vi "Box Colour FGV.vi"(8 "error in (no error)":errorcluster, 10 "Colour to detect":T1=enum."Black", 11 "Init/R/W State":T2) -> (0 "error out":errorcluster, 3 "Colour to detect (output)":T1)   [LabVIEW 2018]
uses:
  Box Colour FGV States.ctl
  Box Colour FGV Colours.ctl
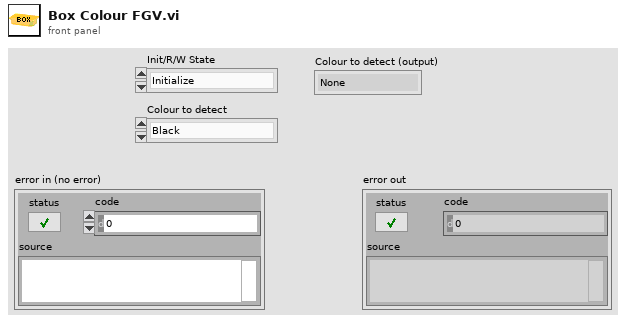
[diagram p1: front panel]
types:
  T1 = typedef "Box Colour FGV Colours.ctl" = enum16{"None", "Black", "Blue", "Green", "Red", "Yellow"}
  T2 = typedef "Box Colour FGV States.ctl" = enum16{"Initialize", "Read", "Write"}
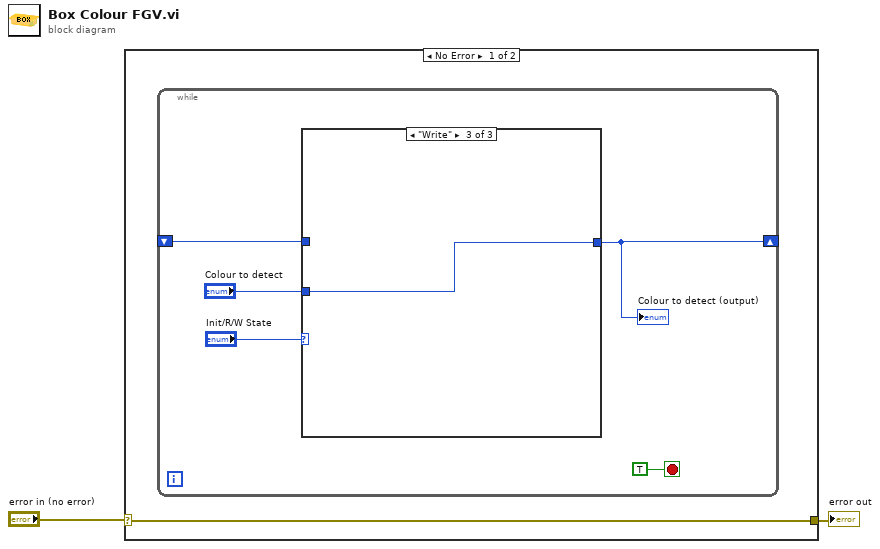
[diagram p0: block diagram]
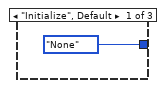
[diagram p2: hidden frame]
diagram:
  n1 = case shown="No Error" "error in (no error)" {
    selector: "error in (no error)" -> [w3 w12]
    tunnel: [w3 w12] -> w1
    frame No Error {
      n2 = while {
        shift-right: [w6] -> _
        shift-left: _ -> [w5]
        stop <- TRUE stop-if-true
        n3 = case shown="\"Write\"" "Init/R/W State" {
          tunnel: [Box_Colour_FGV_Colours."None" ("Colour to detect") w10 w11] -> w6
          tunnel: w5 -> [_ w10 _]
          tunnel: "Colour to detect" -> [_ _ w11]
          frame "Initialize", Default {
          }
          frame "Read" {
          }
          frame "Write" {
          }
        }
        "Colour to detect (output)" <- w6
      }
    }
    frame Error {
    }
  }
  "error out" <- w1
